vi "Direct Registry Edit.vi"() -> ()   [LabVIEW 2014]
uses:
  <vilib>/registry/registry.llb/Registry RtKey.ctl
  <vilib>/registry/registry.llb/Read Registry Value Simple.vi
panel:
  out "String/Binary data":string
  out "error out":errorcluster
  in  "working directory":path=path ""
  out "Error Out":errorcluster
  in  "Error In":errorcluster
  in  "Path to file that needs to be run as admin":path
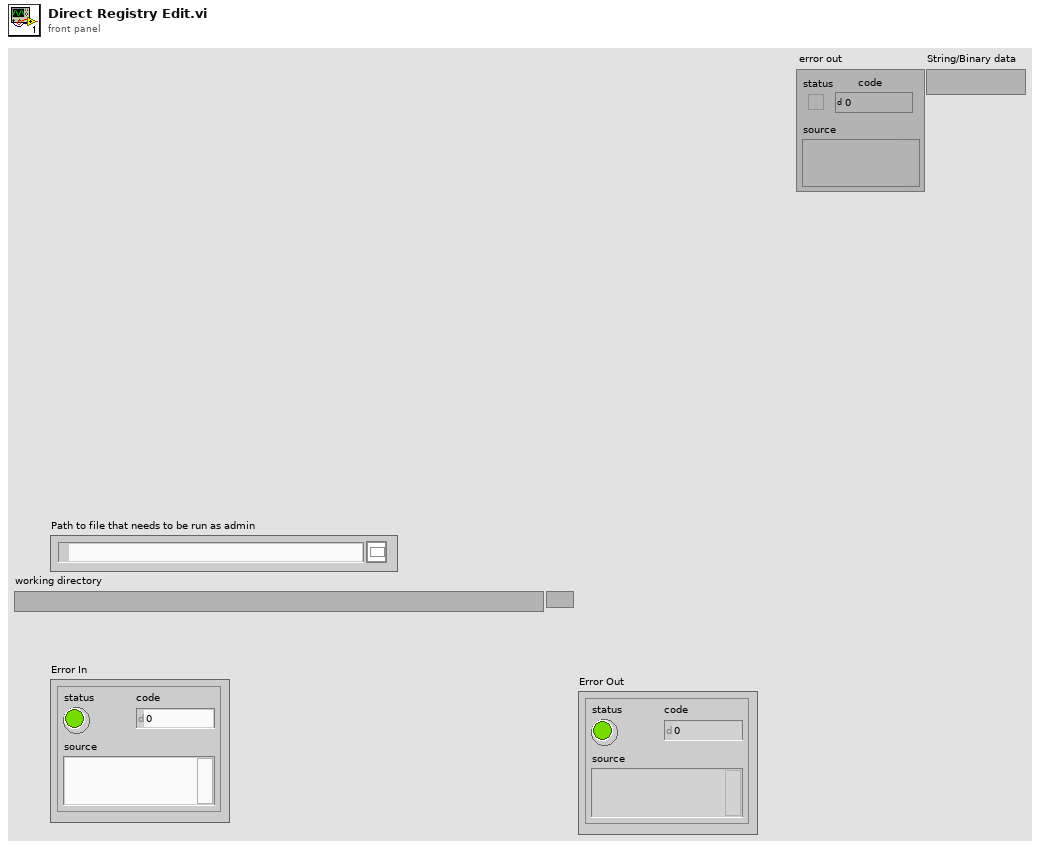
[diagram p1: front panel]
types:
  T1 = typedef "Registry RtKey.ctl" = enum32{"HKEY_CLASSES_ROOT", "HKEY_CURRENT_USER", "HKEY_LOCAL_MACHINE", "HKEY_USERS", "HKEY_PERFORMANCE_DATA", "HKEY_CURRENT_CONFIG", "HKEY_DYN_DATA"}
  T2 = typedef "Registry refnum.ctl" = refnum<k1>
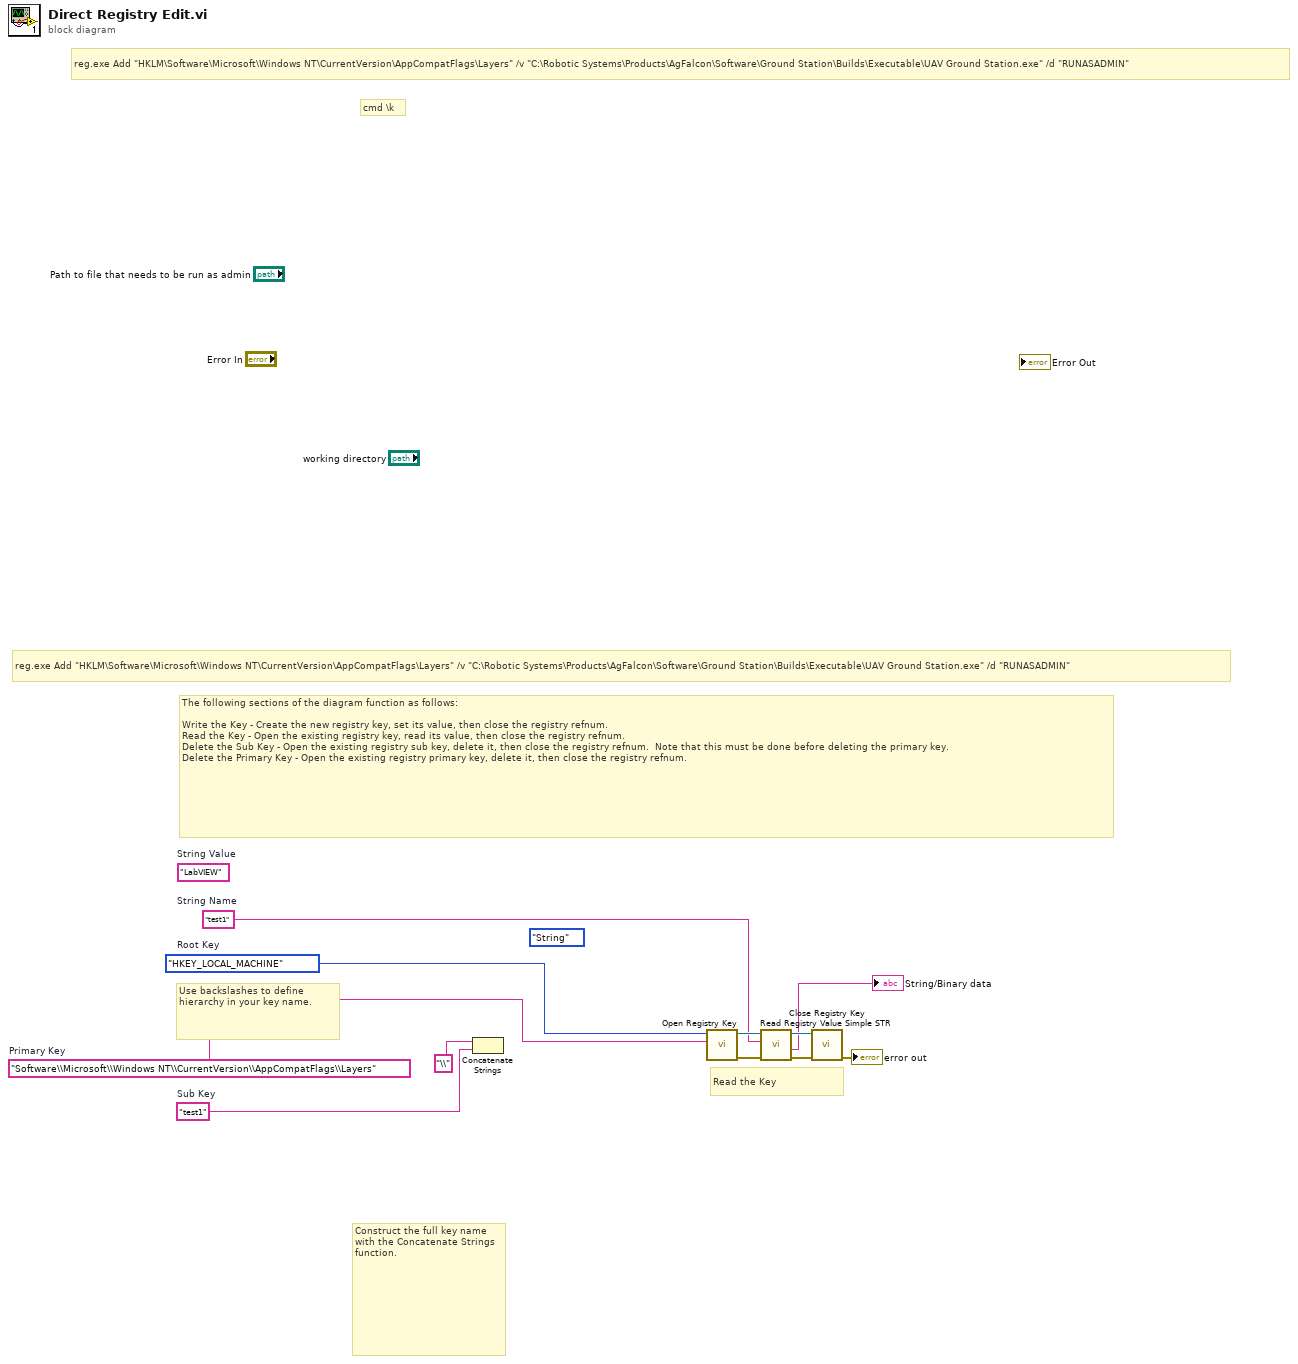
[diagram p0: block diagram]
diagram:
  w6 = "test1"  # Sub Key
  w1 = "Software\\Microsoft\\Windows NT\\CurrentVersion\\AppCompatFlags\\Layers"  # Primary Key
  (unwired) "LabVIEW"  # String Value
  w5 = "test1"  # String Name
  (unwired) enum16{"String", "Binary", "DWORD"}."String" ("simple data type")
  w7 = Registry_RtKey."HKEY_LOCAL_MACHINE"  # Root Key
  # "reg.exe Add \"HKLM\\Software\\Microsoft\\Windows NT\\CurrentVersion\\AppCompatFlags\\Layers\" /v \"C:\\Robotic Systems\\Products\\AgFalcon\\Software\\Ground Station\\Builds\\Executable\\UAV Ground Station.exe\" /d \"RUNASADMIN\""
  # "Construct the full key name with the Concatenate Strings function."
  # "Use backslashes to define hierarchy in your key name."
  # "The following sections of the diagram function as follows:\n\nWrite the Key - Create the new registry key, set its value, then close the registry refnum.\nRead the Key - Open the existing registry key, read its value, then close the registry refnum.\nDelete the Sub Key - Open the existing registry sub key, delete it, then close the registry refnum.  Note that this must be done before deleting the primary key.\nDelete the Primary Key - Open the existing registry primary key, delete it, then close the registry refnum."
  # "Read the Key"
  # "cmd \\k"
  # "reg.exe Add \"HKLM\\Software\\Microsoft\\Windows NT\\CurrentVersion\\AppCompatFlags\\Layers\" /v \"C:\\Robotic Systems\\Products\\AgFalcon\\Software\\Ground Station\\Builds\\Executable\\UAV Ground Station.exe\" /d \"RUNASADMIN\""
  n1 = Concatenate Strings("\\", w6) -> ()  [unwired: 1 out]
  n2 = call <vilib>:"Open Registry Key.vi"("subkey"=w1, "root key (HKEY_LOCAL_MACHINE)"=w7) -> ("error out"=w8:errorcluster, "refnum out"=w9:T2)  [unwired: 8 in]
  n3 = call-poly <vilib>:"Read Registry Value Simple STR.vi"("error in (no error)"=w8, "value"=w5, "refnum"=w9) -> ("error out"=w11:errorcluster, "String/Binary data"=→"String/Binary data":string, "refnum out"=w10:T2)  [unwired: 3 in, 1 out]
  n4 = call <vilib>:"Close Registry Key.vi"("error in (no error)"=w11, "refnum"=w10) -> ("error out"=→"error out":errorcluster)  [unwired: 5 in]
